vi "ToControllerQueue_bac.vi"(7 "Enum":T1, 8 "error in (no error)":errorcluster) -> (0 "error out":errorcluster)   [LabVIEW 2021]
uses:
  QueueEnum.ctl
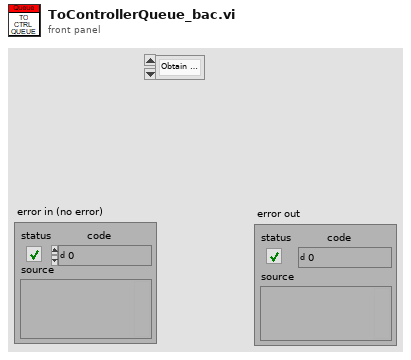
[diagram p1: front panel]
types:
  T1 = typedef "QueueEnum.ctl" = enum16{"Obtain Queue", "Get Queue Ref", "Flush Queue", "Release Queue"}
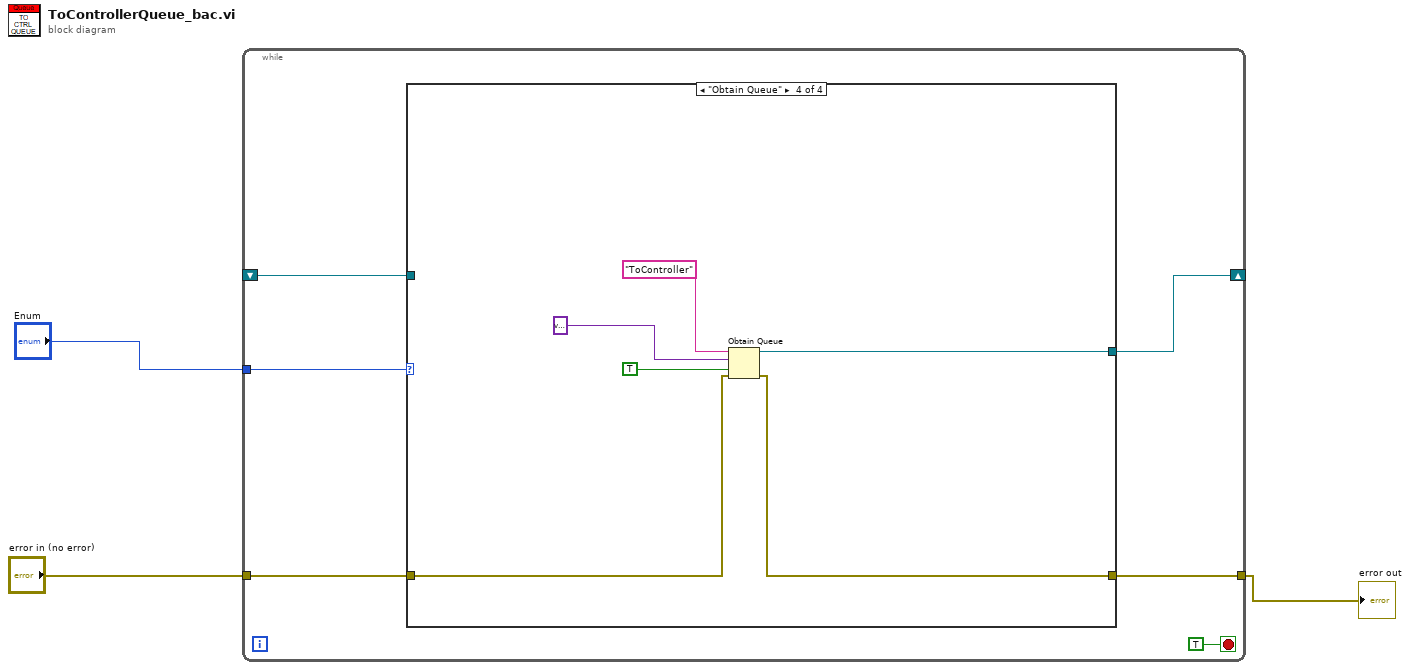
[diagram p0: block diagram]
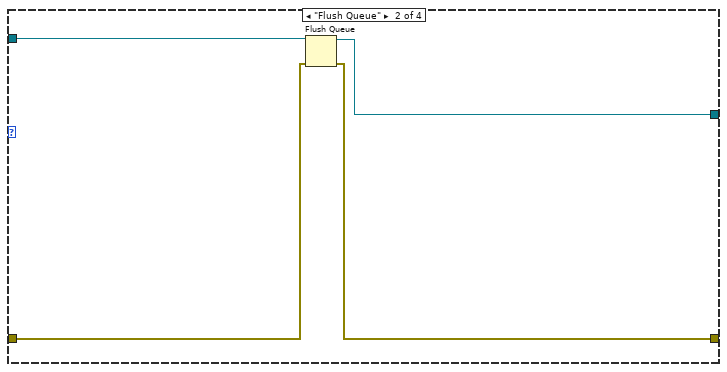
[diagram p3: hidden frame]
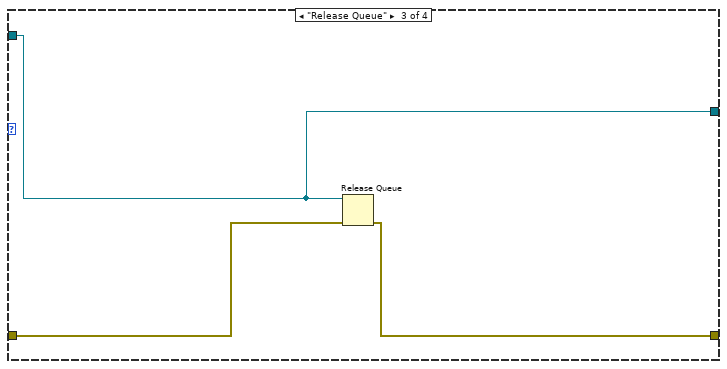
[diagram p4: hidden frame]
diagram:
  n1 = while {
    tunnel: "error in (no error)" -> [w7]
    tunnel: [w6] -> w2
    tunnel: "Enum" -> [w8]
    shift-right: [w5] -> _
    shift-left: _ -> [w4]
    stop <- TRUE stop-if-true
    n2 = case shown="\"Obtain Queue\"" w8 {
      tunnel: w7 -> [w10 w14 w18 w23]
      tunnel: [w10 w13 w17 w21] -> w6
      tunnel: [w11 w12 w16 w20] -> w5
      tunnel: w4 -> [w11 w15 w16 _]
      frame "Get Queue Ref", Default {
      }
      frame "Flush Queue" {
        n3 = Flush Queue(queue=w15, error in (no error)=w14) -> (queue out=w12:refnum<queue>, error out=w13:errorcluster)  [unwired: 1 out]
      }
      frame "Release Queue" {
        n4 = Release Queue(queue=w16, error in (no error)=w18) -> (error out=w17:errorcluster)  [unwired: 1 in, 2 out]
      }
      frame "Obtain Queue" {
        n5 = Obtain Queue(name (unnamed)="ToController", element data type=variant, create if not found? (T)=TRUE, error in (no error)=w23) -> (queue out=w20:refnum<queue>, error out=w21:errorcluster)  [unwired: 1 in, 1 out]
      }
    }
  }
  "error out" <- w2
